vi "Inventory.vi"(8 "error in (no error)":errorcluster, 11 "Productos in":refnum<class "Productos.lvclass">) -> (0 "error out":errorcluster, 2 "Productos 2":T1, 3 "Productos out":refnum<class "Productos.lvclass">)   [LabVIEW 2021, in "Productos.lvlib" / "Productos.lvclass"]
uses:
  Productos.lvclass
  Productos.lvclass/Productos.ctl
panel:
  in  "Productos":T1
  in  "Cancel Button":bool
  in  "OK Button":bool
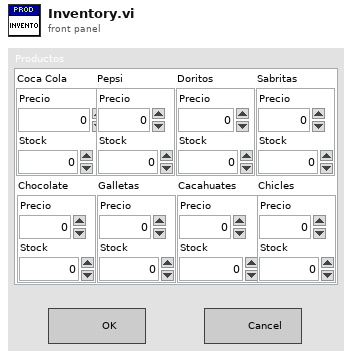
[diagram p1: front panel]
types:
  T1 = cluster{"Coca Cola":cluster{"Precio":dbl, "Stock":dbl}, "Pepsi":cluster{"Precio":dbl, "Stock":dbl}, "Doritos":cluster{"Precio":dbl, "Stock":dbl}, "Sabritas":cluster{"Precio":dbl, "Stock":dbl}, "Chocolate":cluster{"Precio":dbl, "Stock":dbl}, "Galletas":cluster{"Precio":dbl, "Stock":dbl}, "Cacahuates":cluster{"Precio":dbl, "Stock":dbl}, "Chicles":cluster{"Precio":dbl, "Stock":dbl}}
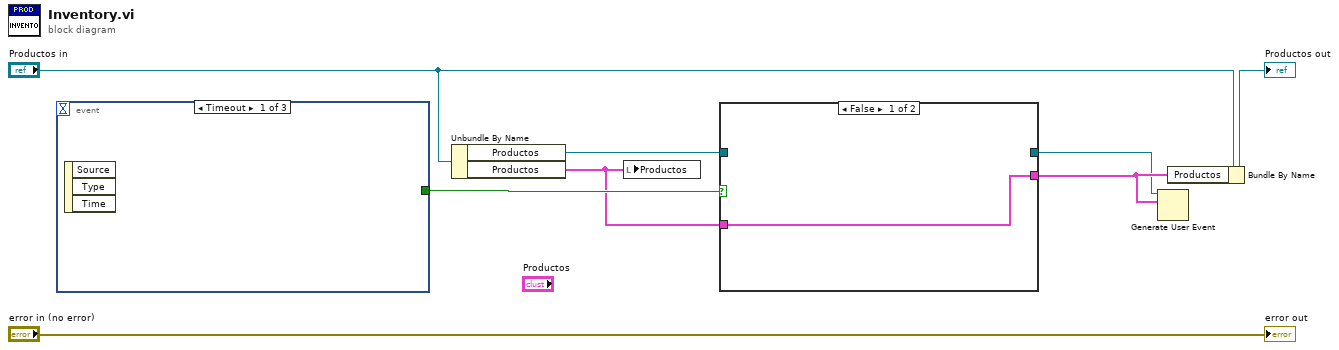
[diagram p0: block diagram]
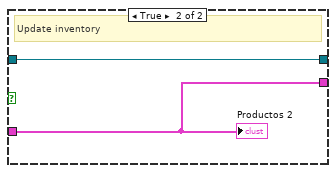
[diagram p2: hidden frame]
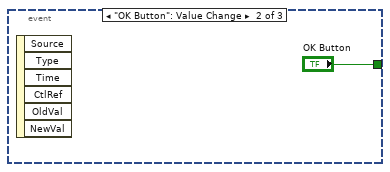
[diagram p3: hidden frame]
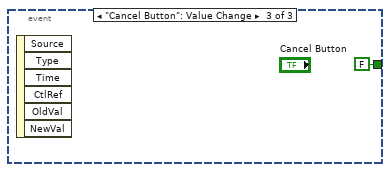
[diagram p4: hidden frame]
diagram:
  n1 = event shown="[0] Timeout" {
    selector: _ -> [_ _ _]
    dyn-events: _ -> [_ _ _]
    timeout: _ -> [_ _ _]
    tunnel: [_ "OK Button" FALSE ("OK Button")] -> w7
    event Timeout {
      n2 = event-data() -> ()  [unwired: 1 in, 3 out]
    }
    event "OK Button": Value Change {
      n3 = event-data() -> ()  [unwired: 1 in, 6 out]
    }
    event "Cancel Button": Value Change {
      n4 = event-data() -> ()  [unwired: 1 in, 6 out]
    }
  }
  n5 = Unbundle By Name("Productos in") -> ("Productos"=w3:refnum<user-event>, "Productos"=w1:T1)
  n6 = local write "Productos"(w1) -> ()
  n7 = case shown="False" w7 {
    tunnel: [w11 w12] -> w4
    tunnel: [_ w13] -> w2
    tunnel: w3 -> [_ w13]
    tunnel: w1 -> [w11 w12]
    frame False {
    }
    frame True {
      # "Update inventory"
      "Productos 2" <- w12
    }
  }
  n8 = Generate User Event(user event=w2, event data cluster=w4) -> ()  [unwired: 2 in, 2 out]
  n9 = Bundle By Name(cluster="Productos in", "Productos"=w4) -> (→"Productos out":refnum<class "Productos.lvclass">)
  "error out" <- "error in (no error)"
